vi "2 - MQTT_Q - GUI.vi"() -> ()   [LabVIEW 2015]
uses:
  src/MQTT_Q.lvclass
panel:
  out "Current Temperature":dbl
  in  "Exit":bool
  in  "Start":bool
  in  "Stop":bool
  in  "Read Temperature interval (ms)":u32=500
  out "Waveform Chart":dbl(graph)
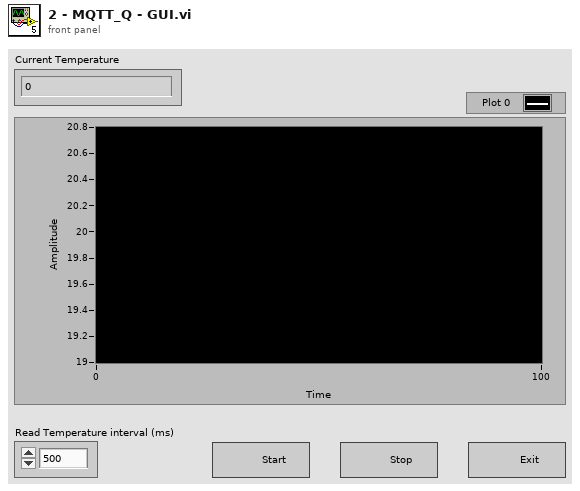
[diagram p1: front panel]
types:
  T1 = cluster{"IP address":string, "Port":u16, "Client ID":string}
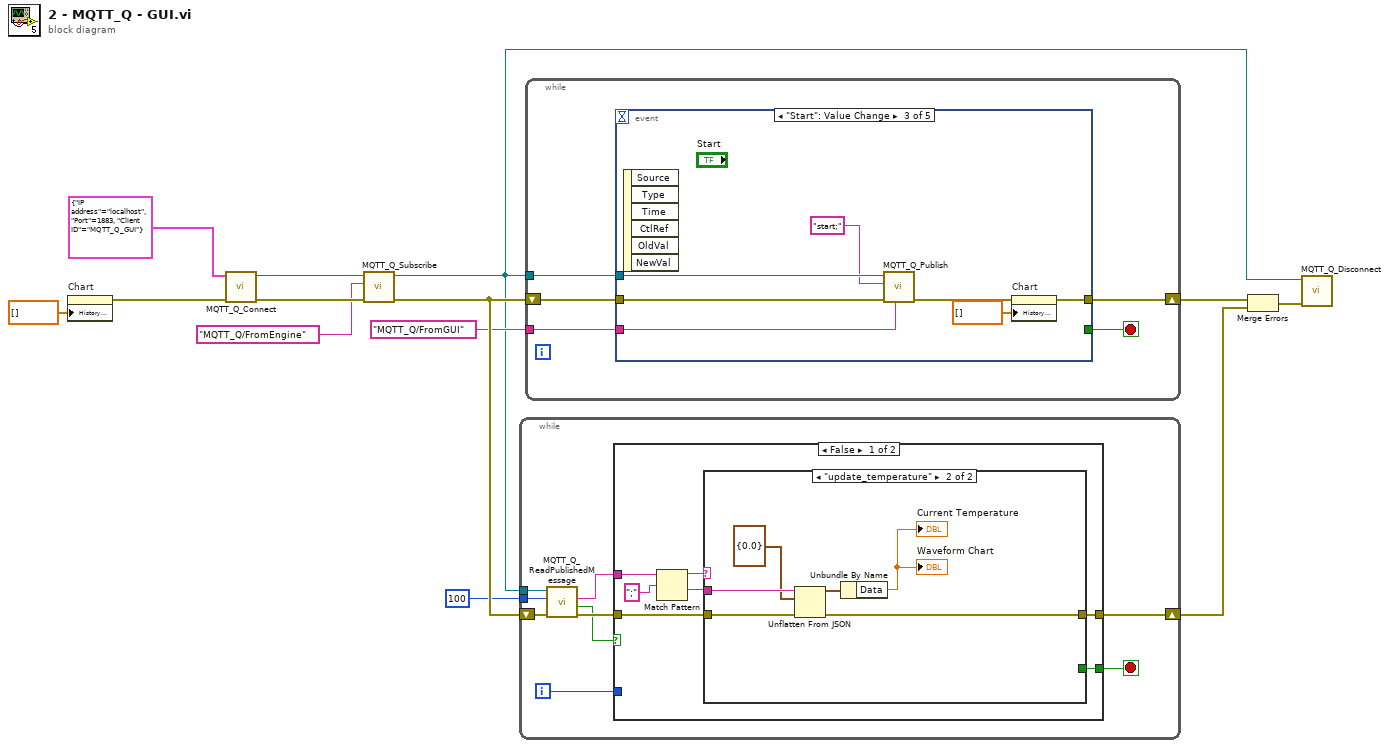
[diagram p0: block diagram]
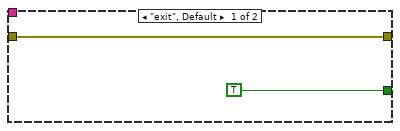
[diagram p2: hidden frame]
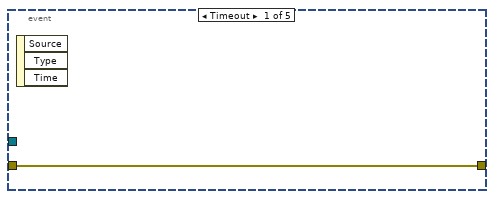
[diagram p4: hidden frame]
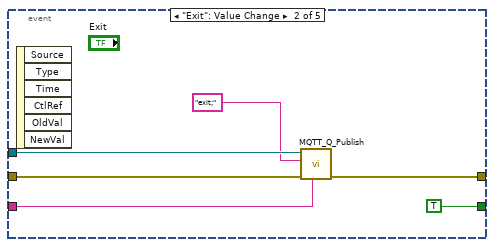
[diagram p5: hidden frame]
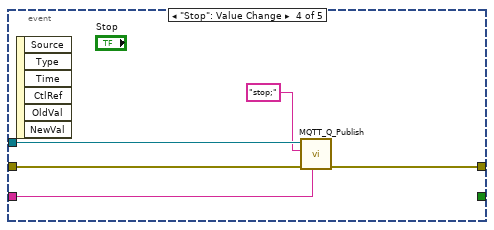
[diagram p6: hidden frame]
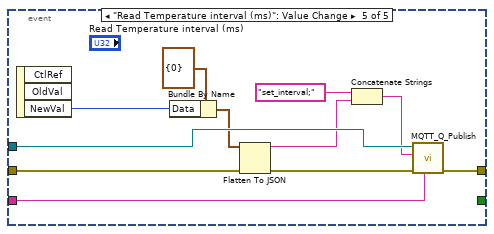
[diagram p7: hidden frame]
diagram:
  n1 = property on="Chart" class="WFChart (strict)"("History Data"=dbl[] []) -> (error out=w9:errorcluster)  [unwired: 2 in, 1 out]
  n2 = call "MQTT_Q_Connect.vi"("error in (no error)"=w9, "MQTT Broker & Client ID"=T1 {"IP address"="localhost", "Port"=1883, "Client ID"="MQTT_Q_GUI"}) -> ("error out"=w11:errorcluster, "MQTT_Q Out"=w10:refnum<class "MQTT_Q.lvclass">)  [unwired: 8 in]
  n3 = call "MQTT_Q_Subscribe.vi"("error in (no error)"=w11, "Topic"="MQTT_Q/FromEngine", "MQTT_Q In"=w10) -> ("error out"=w8:errorcluster, "MQTT_Q Out"=w3:refnum<class "MQTT_Q.lvclass">)  [unwired: 6 in, 1 out]
  n4 = while {
    tunnel: w3 -> [w18]
    shift-right: [w21] -> w6
    shift-left: w8 -> [w20]
    tunnel: 100 ("timeout ms (25000)") -> [w16]
    i -> [w14]
    stop <- w22 stop-if-true
    n5 = call "MQTT_Q_ReadPublishedMessage.vi"("error in (no error)"=w20, "timeout ms (25000)"=w16, "MQTT_Q In"=w18) -> ("error out"=w19:errorcluster, "TimedOut"=w15:bool, "Message"=w17:string)  [unwired: 4 in, 2 out]
    n6 = case shown="False" w15 {
      tunnel: [w29 _] -> w22
      tunnel: [w28 w38] -> w21
      tunnel: w19 -> [w27 w38]
      tunnel: w17 -> [w25 _]
      tunnel: w14 -> [_ _]
      frame False {
        n7 = Match Pattern(string=w25, regular expression=";") -> (before substring=w24:string, after substring=w23:string)  [unwired: 1 in, 2 out]
        n8 = case shown="\"update_temperature\"" w24 {
          tunnel: w27 -> [w30 w37]
          tunnel: [TRUE _] -> w29
          tunnel: w23 -> [_ w35]
          tunnel: [w30 w36] -> w28
          frame "exit", Default {
          }
          frame "update_temperature" {
            n9 = Unflatten From JSON(JSON string=w35, type and defaults=cluster{"Data":dbl} {"Data"=0.0}, error in (no error)=w37) -> (value=w33:cluster{"Data":dbl}, error out=w36:errorcluster)  [unwired: 4 in]
            n10 = Unbundle By Name(w33) -> ("Data"=→"Waveform Chart" →"Current Temperature":dbl)
          }
        }
      }
      frame True {
      }
    }
  }
  n11 = while {
    shift-right: [w41] -> w7
    shift-left: w8 -> [w43]
    tunnel: w3 -> [w42]
    tunnel: "MQTT_Q/FromGUI" ("Topic") -> [w39]
    stop <- w40 stop-if-true
    n12 = event shown="[2] \"Start\": Value Change" {
      selector: _ -> [_ _ _ _ _]
      dyn-events: _ -> [_ _ _ _ _]
      timeout: _ -> [_ _ _ _ _]
      tunnel: w43 -> [w44 w49 w55 w62 w71]
      tunnel: w42 -> [_ w47 w53 w60 w72]
      tunnel: [w44 w48 w56 w61 w73] -> w41
      tunnel: [_ TRUE _ _ _] -> w40
      tunnel: w39 -> [_ w46 w51 w58 w63]
      event Timeout {
        n13 = event-data() -> ()  [unwired: 1 in, 3 out]
      }
      event "Exit": Value Change {
        n14 = event-data() -> ()  [unwired: 1 in, 6 out]
        n15 = call "MQTT_Q_Publish.vi"("Topic"=w46, "error in"=w49, "Message"="exit;" ("Cmd"), "MQTT_Q In"=w47) -> ("error out"=w48:errorcluster)  [unwired: 6 in, 1 out]
      }
      event "Start": Value Change {
        n16 = event-data() -> ()  [unwired: 1 in, 6 out]
        n17 = call "MQTT_Q_Publish.vi"("Topic"=w51, "error in"=w55, "Message"="start;" ("Cmd"), "MQTT_Q In"=w53) -> ("error out"=w54:errorcluster)  [unwired: 6 in, 1 out]
        n18 = property on="Chart" class="WFChart (strict)"(error in=w54, "History Data"=dbl[] []) -> (error out=w56:errorcluster)  [unwired: 1 in, 1 out]
      }
      event "Stop": Value Change {
        n19 = event-data() -> ()  [unwired: 1 in, 6 out]
        n20 = call "MQTT_Q_Publish.vi"("Topic"=w58, "error in"=w62, "Message"="stop;" ("Cmd"), "MQTT_Q In"=w60) -> ("error out"=w61:errorcluster)  [unwired: 6 in, 1 out]
      }
      event "Read Temperature interval (ms)": Value Change {
        n21 = event-data() -> ("NewVal"=w68:u32)  [unwired: 1 in, 2 out]
        n22 = Bundle By Name(cluster=cluster{"Data":u32} {"Data"=0}, "Data"=w68) -> (w67:cluster{"Data":u32})
        n23 = Flatten To JSON(anything=w67, error in (no error)=w71) -> (JSON string=w64:string, 11:w70:errorcluster)  [unwired: 1 in]
        n24 = Concatenate Strings("set_interval;" ("Cmd"), w64) -> (w65:string)
        n25 = call "MQTT_Q_Publish.vi"("Topic"=w63, "error in"=w70, "Message"=w65, "MQTT_Q In"=w72) -> ("error out"=w73:errorcluster)  [unwired: 6 in, 1 out]
      }
    }
  }
  n26 = Merge Errors(w7, w6) -> (w5:errorcluster)
  n27 = call "MQTT_Q_Disconnect.vi"("error in (no error)"=w5, "MQTT_Q In"=w3) -> ()  [unwired: 9 in, 1 out]
